vi "五层电梯.vi"() -> ()   [LabVIEW 2011]
panel:
  in  "上/下行显示":string
  in  "楼层显示":string
  out "电梯内厢显示":string
  out "5层显示":string
  out "4层显示":string
  out "3层显示":string
  out "2层显示":string
  out "1层显示":string
  in  "上/下行控制":i32
  out "内外呼叫数组":bool[](array[boolean])
  out "电梯门":bool
  in  "内呼1层":bool caption="1"
  in  "内呼2层":bool caption="2"
  in  "内呼3层":bool caption="3"
  in  "内呼4层":bool caption="4"
  in  "内呼5层":bool caption="5"
  in  "5下":bool caption="下"
  in  "1上":bool caption="上"
  in  "4下":bool caption="下"
  in  "4上":bool caption="上"
  in  "3下":bool caption="下"
  in  "3上":bool caption="上"
  in  "2下":bool caption="下"
  in  "2上":bool caption="上"
  out "五层门":bool caption="Boolean"
  out "四层门":bool caption="Boolean"
  out "三层门":bool caption="Boolean"
  out "二层门":bool caption="Boolean"
  out "一层门":bool caption="Boolean"
  out "电梯":bool
  # "五层电梯示意图"
  # "5"
  # "4"
  # "3"
  # "电梯内厢"
  # "2"
  # "1"
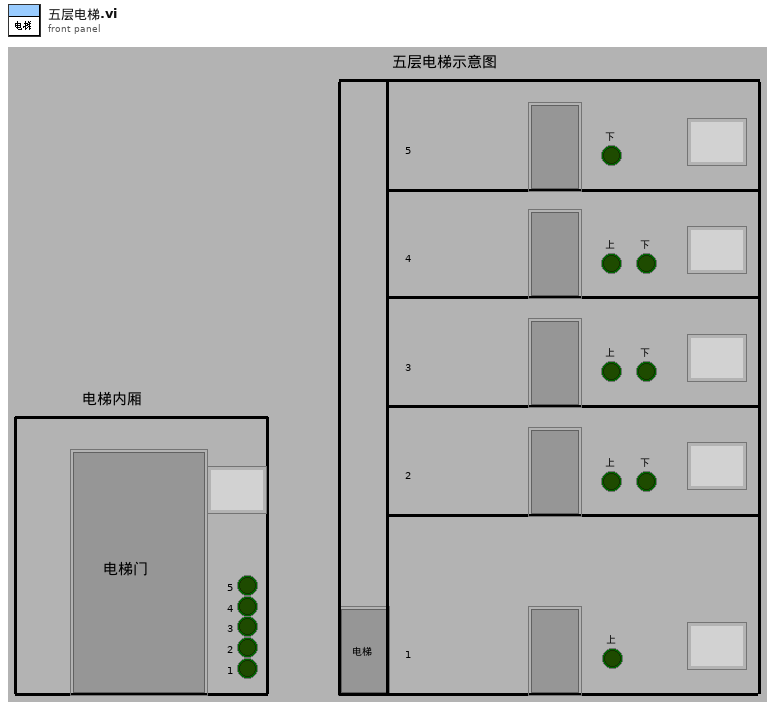
[diagram p1: front panel]
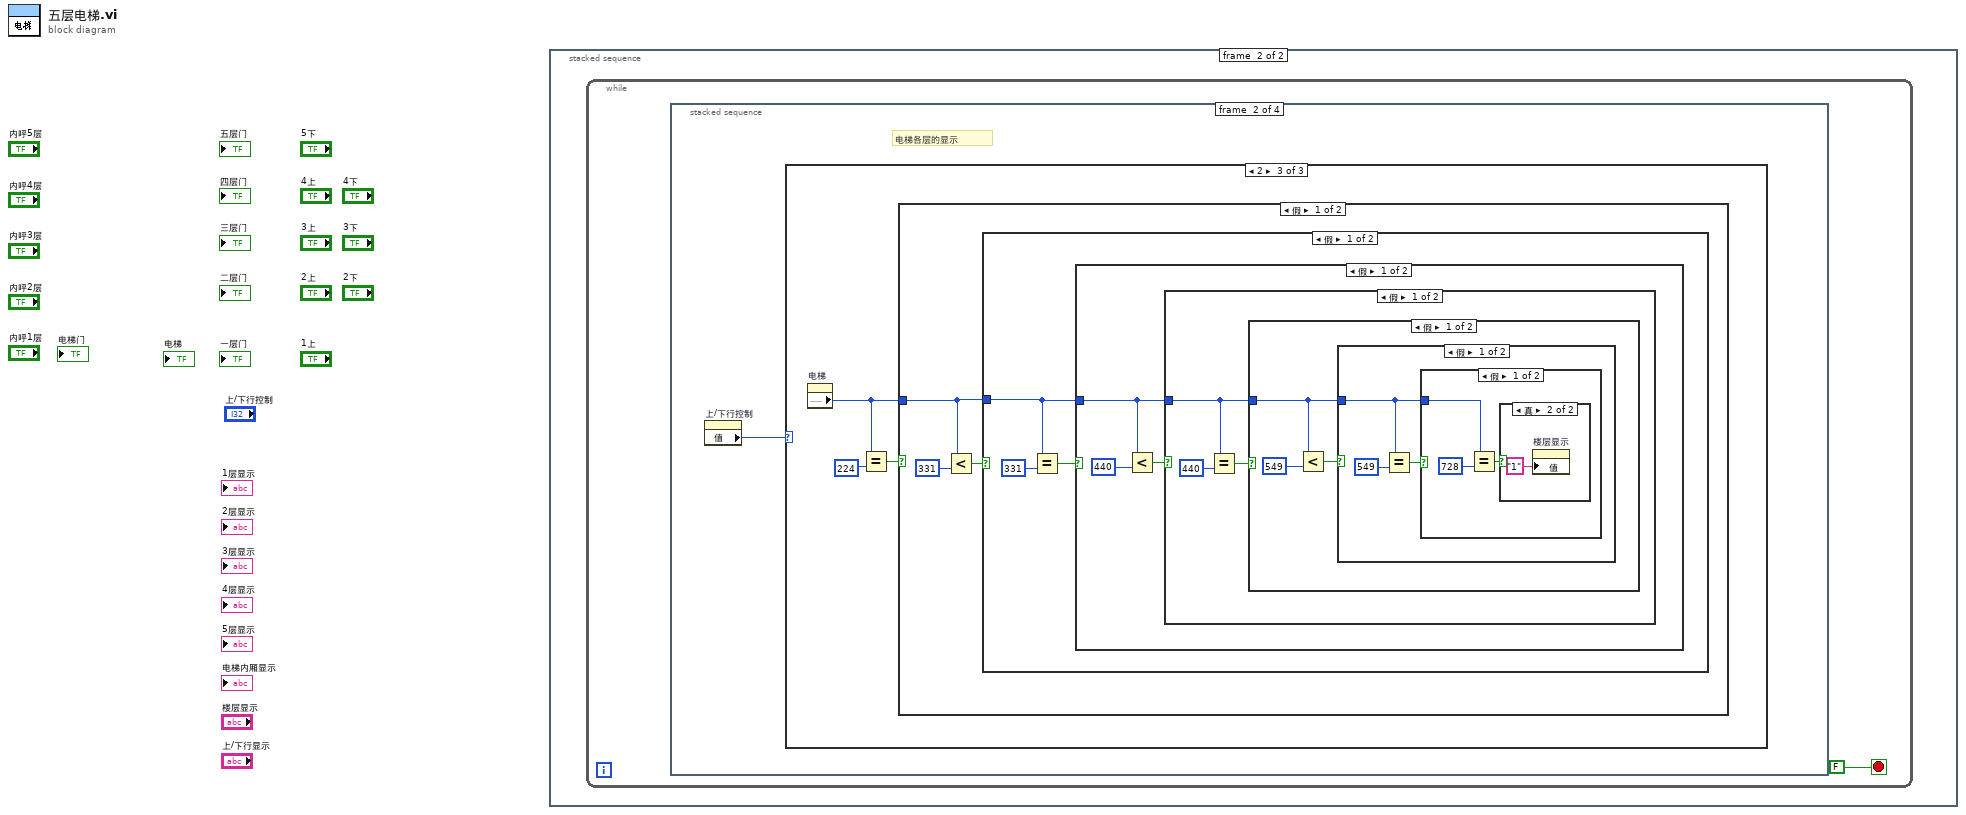
[diagram p0: block diagram]
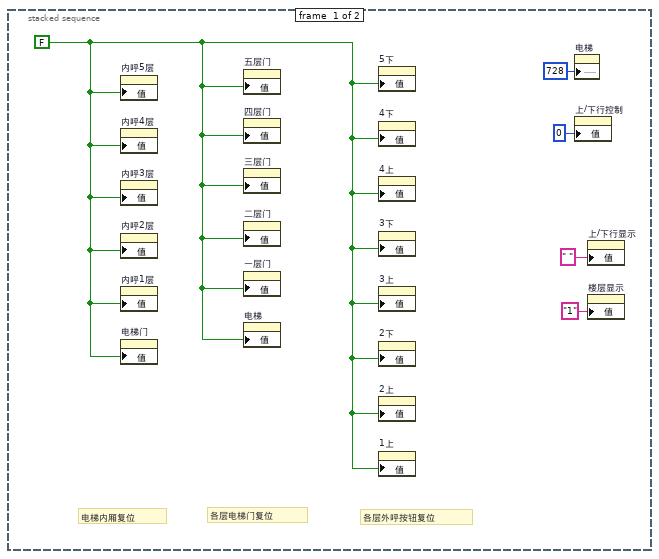
[diagram p2: hidden frame]
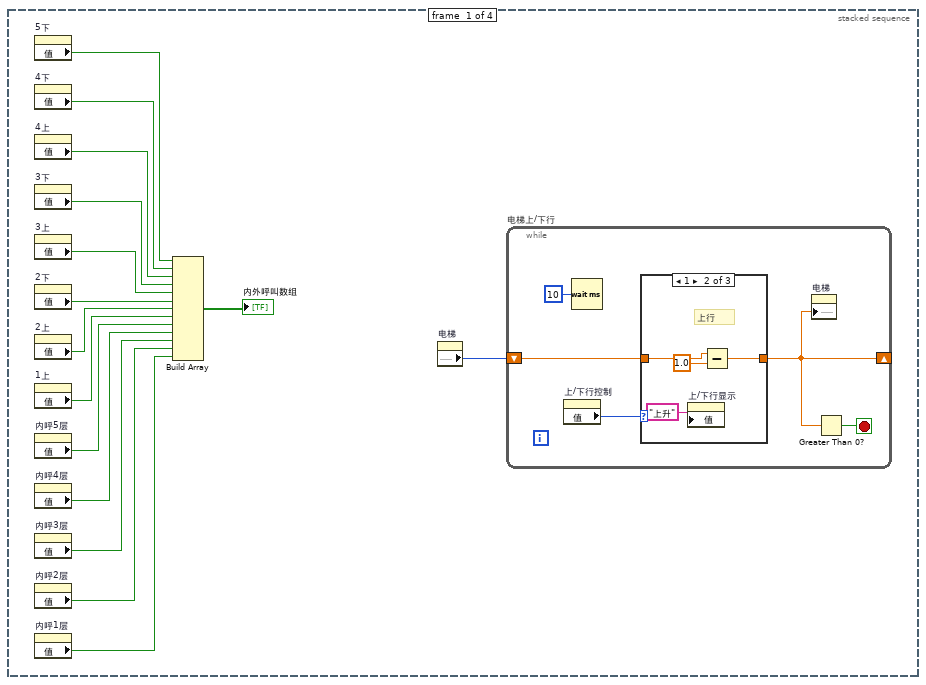
[diagram p3: hidden frame]
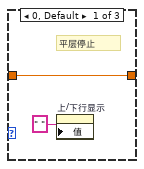
[diagram p4: hidden frame]
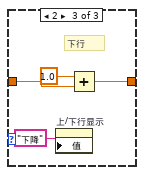
[diagram p5: hidden frame]
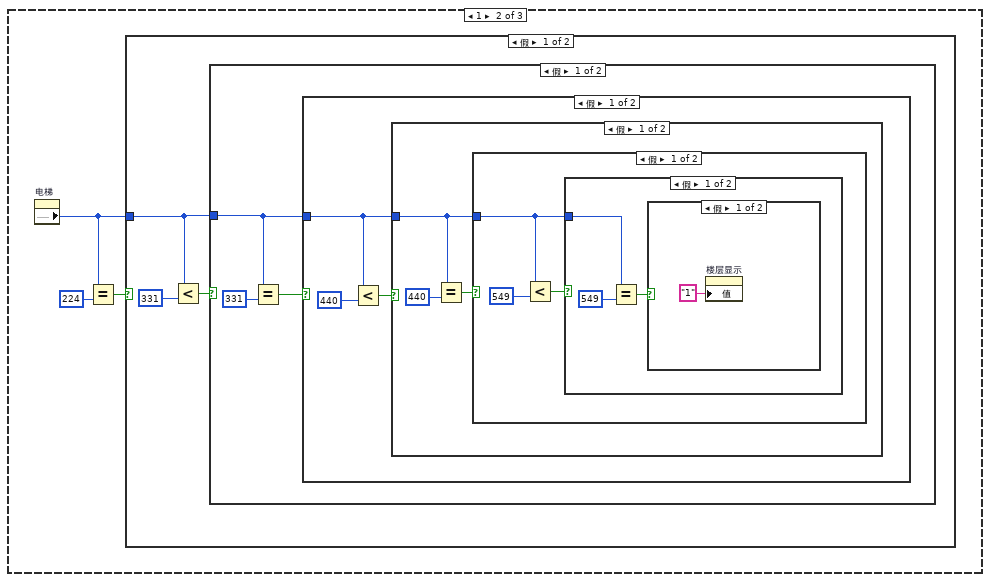
[diagram p7: hidden frame]
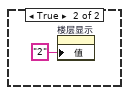
[diagram p8: hidden frame]
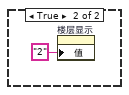
[diagram p9: hidden frame]
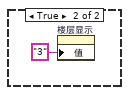
[diagram p10: hidden frame]
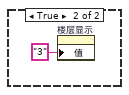
[diagram p11: hidden frame]
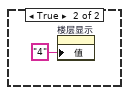
[diagram p12: hidden frame]
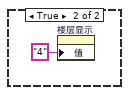
[diagram p13: hidden frame]
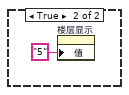
[diagram p14: hidden frame]
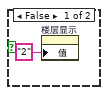
[diagram p15: hidden frame]
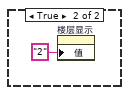
[diagram p16: hidden frame]
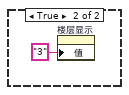
[diagram p17: hidden frame]
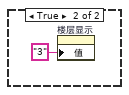
[diagram p18: hidden frame]
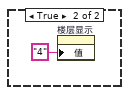
[diagram p19: hidden frame]
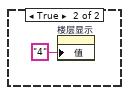
[diagram p20: hidden frame]
diagram:
  n1 = stacked-sequence {
    frame #0 {
      w3 = FALSE ("开门")
      # "各层外呼按钮复位"
      # "各层电梯门复位"
      # "电梯内厢复位"
      n2 = property on="内呼5层" class="Bool (严格)"("值"=w3) -> ()  [unwired: 2 in, 2 out]
      n3 = property on="内呼4层" class="Bool (严格)"("值"=w3) -> ()  [unwired: 2 in, 2 out]
      n4 = property on="内呼3层" class="Bool (严格)"("值"=w3) -> ()  [unwired: 2 in, 2 out]
      n5 = property on="内呼2层" class="Bool (严格)"("值"=w3) -> ()  [unwired: 2 in, 2 out]
      n6 = property on="内呼1层" class="Bool (严格)"("值"=w3) -> ()  [unwired: 2 in, 2 out]
      n7 = property on="电梯门" class="Bool (严格)"("值"=w3) -> ()  [unwired: 2 in, 2 out]
      n8 = property on="五层门" class="Bool (严格)"("值"=w3) -> ()  [unwired: 2 in, 2 out]
      n9 = property on="四层门" class="Bool (严格)"("值"=w3) -> ()  [unwired: 2 in, 2 out]
      n10 = property on="三层门" class="Bool (严格)"("值"=w3) -> ()  [unwired: 2 in, 2 out]
      n11 = property on="二层门" class="Bool (严格)"("值"=w3) -> ()  [unwired: 2 in, 2 out]
      n12 = property on="一层门" class="Bool (严格)"("值"=w3) -> ()  [unwired: 2 in, 2 out]
      n13 = property on="电梯" class="Bool (严格)"("值"=w3) -> ()  [unwired: 2 in, 2 out]
      n14 = property on="5下" class="Bool (严格)"("值"=w3) -> ()  [unwired: 2 in, 2 out]
      n15 = property on="4下" class="Bool (严格)"("值"=w3) -> ()  [unwired: 2 in, 2 out]
      n16 = property on="4上" class="Bool (严格)"("值"=w3) -> ()  [unwired: 2 in, 2 out]
      n17 = property on="3下" class="Bool (严格)"("值"=w3) -> ()  [unwired: 2 in, 2 out]
      n18 = property on="3上" class="Bool (严格)"("值"=w3) -> ()  [unwired: 2 in, 2 out]
      n19 = property on="2下" class="Bool (严格)"("值"=w3) -> ()  [unwired: 2 in, 2 out]
      n20 = property on="2上" class="Bool (严格)"("值"=w3) -> ()  [unwired: 2 in, 2 out]
      n21 = property on="1上" class="Bool (严格)"("值"=w3) -> ()  [unwired: 2 in, 2 out]
      n22 = property on="电梯" class="Bool (严格)"("位置:置顶"=728 ("Position:Top")) -> ()  [unwired: 2 in, 2 out]
      n23 = property on="上/下行控制" class="DigNum (严格)"("值"=0 ("上/下行控制")) -> ()  [unwired: 2 in, 2 out]
      n24 = property on="上/下行显示" class="Str"("值"=" " ("上/下行显示")) -> ()  [unwired: 2 in, 2 out]
      n25 = property on="楼层显示" class="Str"("值"="1" ("楼层显示")) -> ()  [unwired: 2 in, 2 out]
    }
    frame #1 {
      n26 = while {
        stop <- FALSE stop-if-true
        n27 = stacked-sequence {
          frame #0 {
            n28 = property on="5下" class="Bool (严格)"() -> ("值"=w20:bool)  [unwired: 2 in, 2 out]
            n29 = property on="4下" class="Bool (严格)"() -> ("值"=w19:bool)  [unwired: 2 in, 2 out]
            n30 = property on="4上" class="Bool (严格)"() -> ("值"=w18:bool)  [unwired: 2 in, 2 out]
            n31 = property on="3下" class="Bool (严格)"() -> ("值"=w17:bool)  [unwired: 2 in, 2 out]
            n32 = property on="3上" class="Bool (严格)"() -> ("值"=w16:bool)  [unwired: 2 in, 2 out]
            n33 = property on="2下" class="Bool (严格)"() -> ("值"=w15:bool)  [unwired: 2 in, 2 out]
            n34 = property on="2上" class="Bool (严格)"() -> ("值"=w14:bool)  [unwired: 2 in, 2 out]
            n35 = property on="1上" class="Bool (严格)"() -> ("值"=w13:bool)  [unwired: 2 in, 2 out]
            n36 = property on="内呼5层" class="Bool (严格)"() -> ("值"=w12:bool)  [unwired: 2 in, 2 out]
            n37 = property on="内呼4层" class="Bool (严格)"() -> ("值"=w11:bool)  [unwired: 2 in, 2 out]
            n38 = property on="内呼3层" class="Bool (严格)"() -> ("值"=w10:bool)  [unwired: 2 in, 2 out]
            n39 = property on="内呼2层" class="Bool (严格)"() -> ("值"=w9:bool)  [unwired: 2 in, 2 out]
            n40 = property on="内呼1层" class="Bool (严格)"() -> ("值"=w8:bool)  [unwired: 2 in, 2 out]
            n41 = Build Array(w20, w19, w18, w17, w16, w15, w14, w13, w12, w11, w10, w9, w8) -> (→"内外呼叫数组":bool[])
            n42 = property on="电梯" class="Bool (严格)"() -> ("位置:置顶"=w21:i32)  [unwired: 2 in, 2 out]
            n43 = while "电梯上/下行" {
              shift-right: [w23] -> _
              shift-left: w21 -> [w24]
              stop <- w22 stop-if-true
              n44 = property on="上/下行控制" class="DigNum (严格)"() -> ("值"=w25:i32)  [unwired: 2 in, 2 out]
              n45 = Wait (ms)(milliseconds to wait=u32 10) -> ()  [unwired: 1 out]
              n46 = case shown="1" w25 {
                tunnel: w24 -> [w28 w31 w36]
                tunnel: [w28 w32 w35] -> w23
                frame 0, Default {
                  # "平层停止"
                  n47 = property on="上/下行显示" class="Str"("值"=" " ("上/下行显示")) -> ()  [unwired: 2 in, 2 out]
                }
                frame 1 {
                  # "上行"
                  n48 = property on="上/下行显示" class="Str"("值"="上升" ("上/下行显示")) -> ()  [unwired: 2 in, 2 out]
                  n49 = Subtract(x=w31, y=1.0) -> (x-y=w32:dbl)
                }
                frame 2 {
                  # "下行"
                  n50 = property on="上/下行显示" class="Str"("值"="下降" ("上/下行显示")) -> ()  [unwired: 2 in, 2 out]
                  n51 = Add(x=1.0, y=w36) -> (x+y=w35:dbl)
                }
              }
              n52 = property on="电梯" class="Bool (严格)"("位置:置顶"=w23) -> ()  [unwired: 2 in, 2 out]
              n53 = Greater Than 0?(x=w23) -> (x > 0?=w22:bool)
            }
          }
          frame #1 {
            # "电梯各层的显示"
            n54 = property on="上/下行控制" class="DigNum (严格)"() -> ("值"=w37:i32)  [unwired: 2 in, 2 out]
            n55 = case shown="2" w37 {
              frame 0, Default {
              }
              frame 1 {
                n56 = property on="电梯" class="Bool (严格)"() -> ("位置:置顶"=w38:i32)  [unwired: 2 in, 2 out]
                n57 = Equal?(x=w38, y=224) -> (x = y?=w39:bool)
                n58 = case shown="假" w39 {
                  tunnel: w38 -> [w41 _]
                  frame False {
                    n59 = Less?(x=w41, y=331) -> (x < y?=w42:bool)
                    n60 = case shown="假" w42 {
                      tunnel: w41 -> [w44 _]
                      frame False {
                        n61 = Equal?(x=w44, y=331) -> (x = y?=w45:bool)
                        n62 = case shown="假" w45 {
                          tunnel: w44 -> [w47 _]
                          frame False {
                            n63 = Less?(x=w47, y=440) -> (x < y?=w48:bool)
                            n64 = case shown="假" w48 {
                              tunnel: w47 -> [w50 _]
                              frame False {
                                n65 = Equal?(x=w50, y=440) -> (x = y?=w51:bool)
                                n66 = case shown="假" w51 {
                                tunnel: w50 -> [w53 _]
                                frame False {
                                n67 = Less?(x=w53, y=549) -> (x < y?=w54:bool)
                                n68 = case shown="假" w54 {
                                tunnel: w53 -> [w57 _]
                                frame False {
                                n69 = Equal?(x=w57, y=549) -> (x = y?=w56:bool)
                                n70 = case shown="假" w56 {
                                frame False {
                                n71 = property on="楼层显示" class="Str"("值"="1" ("楼层显示")) -> ()  [unwired: 2 in, 2 out]
                                }
                                frame True {
                                n72 = property on="楼层显示" class="Str"("值"="2" ("楼层显示")) -> ()  [unwired: 2 in, 2 out]
                                }
                                }
                                }
                                frame True {
                                n73 = property on="楼层显示" class="Str"("值"="2" ("楼层显示")) -> ()  [unwired: 2 in, 2 out]
                                }
                                }
                                }
                                frame True {
                                n74 = property on="楼层显示" class="Str"("值"="3" ("楼层显示")) -> ()  [unwired: 2 in, 2 out]
                                }
                                }
                              }
                              frame True {
                                n75 = property on="楼层显示" class="Str"("值"="3" ("楼层显示")) -> ()  [unwired: 2 in, 2 out]
                              }
                            }
                          }
                          frame True {
                            n76 = property on="楼层显示" class="Str"("值"="4" ("楼层显示")) -> ()  [unwired: 2 in, 2 out]
                          }
                        }
                      }
                      frame True {
                        n77 = property on="楼层显示" class="Str"("值"="4" ("楼层显示")) -> ()  [unwired: 2 in, 2 out]
                      }
                    }
                  }
                  frame True {
                    n78 = property on="楼层显示" class="Str"("值"="5" ("楼层显示")) -> ()  [unwired: 2 in, 2 out]
                  }
                }
              }
              frame 2 {
                n79 = property on="电梯" class="Bool (严格)"() -> ("位置:置顶"=w67:i32)  [unwired: 2 in, 2 out]
                n80 = Equal?(x=w67, y=224) -> (x = y?=w68:bool)
                n81 = case shown="假" w68 {
                  tunnel: w67 -> [w70 _]
                  frame False {
                    n82 = Less?(x=w70, y=331) -> (x < y?=w71:bool)
                    n83 = case shown="假" w71 {
                      tunnel: w70 -> [w73 _]
                      frame False {
                        n84 = Equal?(x=w73, y=331) -> (x = y?=w74:bool)
                        n85 = case shown="假" w74 {
                          tunnel: w73 -> [w76 _]
                          frame False {
                            n86 = Less?(x=w76, y=440) -> (x < y?=w77:bool)
                            n87 = case shown="假" w77 {
                              tunnel: w76 -> [w79 _]
                              frame False {
                                n88 = Equal?(x=w79, y=440) -> (x = y?=w80:bool)
                                n89 = case shown="假" w80 {
                                tunnel: w79 -> [w82 _]
                                frame False {
                                n90 = Less?(x=w82, y=549) -> (x < y?=w83:bool)
                                n91 = case shown="假" w83 {
                                tunnel: w82 -> [w85 _]
                                frame False {
                                n92 = Equal?(x=w85, y=549) -> (x = y?=w86:bool)
                                n93 = case shown="假" w86 {
                                tunnel: w85 -> [w89 _]
                                frame False {
                                n94 = Equal?(x=w89, y=728) -> (x = y?=w88:bool)
                                n95 = case shown="真" w88 {
                                frame False {
                                n96 = property on="楼层显示" class="Str"("值"="2" ("楼层显示")) -> ()  [unwired: 2 in, 2 out]
                                }
                                frame True {
                                n97 = property on="楼层显示" class="Str"("值"="1" ("楼层显示")) -> ()  [unwired: 2 in, 2 out]
                                }
                                }
                                }
                                frame True {
                                n98 = property on="楼层显示" class="Str"("值"="2" ("楼层显示")) -> ()  [unwired: 2 in, 2 out]
                                }
                                }
                                }
                                frame True {
                                n99 = property on="楼层显示" class="Str"("值"="3" ("楼层显示")) -> ()  [unwired: 2 in, 2 out]
                                }
                                }
                                }
                                frame True {
                                n100 = property on="楼层显示" class="Str"("值"="3" ("楼层显示")) -> ()  [unwired: 2 in, 2 out]
                                }
                                }
                              }
                              frame True {
                                n101 = property on="楼层显示" class="Str"("值"="4" ("楼层显示")) -> ()  [unwired: 2 in, 2 out]
                              }
                            }
                          }
                          frame True {
                            n102 = property on="楼层显示" class="Str"("值"="4" ("楼层显示")) -> ()  [unwired: 2 in, 2 out]
                          }
                        }
                      }
                      frame True {
                        n103 = property on="楼层显示" class="Str"("值"="5" ("楼层显示")) -> ()  [unwired: 2 in, 2 out]
                      }
                    }
                  }
                  frame True {
                    n104 = property on="楼层显示" class="Str"("值"="5" ("楼层显示")) -> ()  [unwired: 2 in, 2 out]
                  }
                }
              }
            }
          }
          frame #2 {
            n105 = property on="上/下行显示" class="Str"() -> ("值"=w101:string)  [unwired: 2 in, 2 out]
            n106 = property on="楼层显示" class="Str"() -> ("值"=w103:string)  [unwired: 2 in, 2 out]
            n107 = Concatenate Strings(w101, "\r", w103) -> (w100:string)
            n108 = property on="1层显示" class="Str"("值"=w100) -> ()  [unwired: 2 in, 2 out]
            n109 = property on="2层显示" class="Str"("值"=w100) -> ()  [unwired: 2 in, 2 out]
            n110 = property on="3层显示" class="Str"("值"=w100) -> ()  [unwired: 2 in, 2 out]
            n111 = property on="4层显示" class="Str"("值"=w100) -> ()  [unwired: 2 in, 2 out]
            n112 = property on="5层显示" class="Str"("值"=w100) -> ()  [unwired: 2 in, 2 out]
            n113 = property on="电梯内厢显示" class="Str"("值"=w100) -> ()  [unwired: 2 in, 2 out]
          }
          frame #3 {
            n114 = property on="电梯" class="Bool (严格)"() -> ("位置:置顶"=w104:i32)  [unwired: 2 in, 2 out]
            n115 = case shown="440" w104 {
              frame 0, Default {
              }
              frame 728 {
                # "一层动作"
                n116 = stacked-sequence {
                  frame #0 {
                    n117 = property on="内呼1层" class="Bool (严格)"() -> ("值"=w107:bool)  [unwired: 2 in, 2 out]
                    n118 = property on="1上" class="Bool (严格)"() -> ("值"=w106:bool)  [unwired: 2 in, 2 out]
                    n119 = Or(x=w107, y=w106) -> (x .or. y?=w105:bool)
                    n120 = case shown="假" w105 {
                      frame False {
                      }
                      frame True {
                        n121 = stacked-sequence {
                          frame #0 {
                            w108 = TRUE ("一层门")
                            # "开门"
                            n122 = property on="一层门" class="Bool (严格)"("值"=w108) -> ()  [unwired: 2 in, 2 out]
                            n123 = property on="电梯门" class="Bool (严格)"("值"=w108) -> ()  [unwired: 2 in, 2 out]
                          }
                          frame #1 {
                            # "进出电梯延时"
                            n124 = Wait (ms)(milliseconds to wait=u32 3000) -> ()  [unwired: 1 out]
                          }
                          frame #2 {
                            w110 = FALSE ("一层门")
                            # "关门"
                            n125 = property on="内呼1层" class="Bool (严格)"("值"=w110) -> ()  [unwired: 2 in, 2 out]
                            n126 = property on="1上" class="Bool (严格)"("值"=w110) -> ()  [unwired: 2 in, 2 out]
                            n127 = property on="一层门" class="Bool (严格)"("值"=w110) -> ()  [unwired: 2 in, 2 out]
                            n128 = property on="电梯门" class="Bool (严格)"("值"=w110) -> ()  [unwired: 2 in, 2 out]
                          }
                        }
                      }
                    }
                  }
                  frame #1 {
                    n129 = property on="内外呼叫数组" class="Arr (严格)"() -> ("值"=w125:bool[])  [unwired: 2 in, 2 out]
                    n130 = Index Array(array=w125, index #1=0 ("index"), index #8=8 ("index")) -> (element #1=w122:bool, element #2=w121:bool, element #3=w120:bool, element #4=w119:bool, element #5=w118:bool, element #6=w117:bool, element #7=w116:bool, element #8=w115:bool, element #9=w114:bool, element #10=w113:bool, element #11=w112:bool)  [unwired: 9 in]
                    n131 = Build Array(w122, w121, w120, w119, w118, w117, w116, w115, w114, w113, w112) -> (w111:bool[])
                    n132 = Or Array Elements(Boolean array=w111) -> (logical OR=w126:bool)
                    n133 = case shown="真" w126 {
                      frame False {
                        n134 = property on="上/下行控制" class="DigNum (严格)"("值"=0 ("上/下行控制")) -> ()  [unwired: 2 in, 2 out]
                      }
                      frame True {
                        n135 = property on="上/下行控制" class="DigNum (严格)"("值"=1 ("上/下行控制")) -> ()  [unwired: 2 in, 2 out]
                      }
                    }
                  }
                }
              }
              frame 549 {
                # "二层动作"
                n136 = property on="上/下行控制" class="DigNum (严格)"() -> ("值"=w129:i32)  [unwired: 2 in, 2 out]
                n137 = case shown="1" w129 {
                  frame 0, Default {
                    # "从静止到上行，下行，同时响应时采取就近原则"
                    n138 = stacked-sequence {
                      frame #0 {
                        # "二层开关门动作"
                        n139 = property on="内外呼叫数组" class="Arr (严格)"() -> ("值"=w132:bool[])  [unwired: 2 in, 2 out]
                        n140 = Index Array(array=w132, index #1=5 ("index"), index #3=11 ("index")) -> (element #1=w134:bool, element #2=w135:bool, element #3=w136:bool)  [unwired: 1 in]
                        n141 = Build Array(w134, w135, w136) -> (w137:bool[])
                        n142 = Or Array Elements(Boolean array=w137) -> (logical OR=w130:bool)
                        n143 = case shown="真" w130 {
                          frame False {
                          }
                          frame True {
                            n144 = stacked-sequence {
                              frame #0 {
                                w138 = TRUE ("二层门")
                                # "开门"
                                n145 = property on="二层门" class="Bool (严格)"("值"=w138) -> ()  [unwired: 2 in, 2 out]
                                n146 = property on="电梯门" class="Bool (严格)"("值"=w138) -> ()  [unwired: 2 in, 2 out]
                              }
                              frame #1 {
                                # "进出电梯延时"
                                n147 = Wait (ms)(milliseconds to wait=u32 3000) -> ()  [unwired: 1 out]
                              }
                              frame #2 {
                                w140 = FALSE ("二层门")
                                # "关门"
                                n148 = property on="2下" class="Bool (严格)"("值"=w140) -> ()  [unwired: 2 in, 2 out]
                                n149 = property on="二层门" class="Bool (严格)"("值"=w140) -> ()  [unwired: 2 in, 2 out]
                                n150 = property on="电梯门" class="Bool (严格)"("值"=w140) -> ()  [unwired: 2 in, 2 out]
                                n151 = property on="2上" class="Bool (严格)"("值"=w140) -> ()  [unwired: 2 in, 2 out]
                                n152 = property on="内呼2层" class="Bool (严格)"("值"=w140) -> ()  [unwired: 2 in, 2 out]
                              }
                            }
                          }
                        }
                      }
                      frame #1 {
                        n153 = property on="内外呼叫数组" class="Arr (严格)"() -> ("值"=w146:bool[])  [unwired: 2 in, 2 out]
                        n154 = Index Array(array=w146, index #1=0 ("index"), index #6=8 ("index")) -> (element #1=w148:bool, element #2=w149:bool, element #3=w150:bool, element #4=w151:bool, element #5=w152:bool, element #6=w143:bool, element #7=w142:bool, element #8=w141:bool)  [unwired: 6 in]
                        n155 = Build Array(w148, w149, w150, w151, w152, w143, w142, w141) -> (w153:bool[])
                        n156 = Or Array Elements(Boolean array=w153) -> (logical OR=w145:bool)
                        n157 = case shown="真" w145 {
                          frame False {
                          }
                          frame True {
                            n158 = property on="上/下行控制" class="DigNum (严格)"("值"=1 ("上/下行控制")) -> ()  [unwired: 2 in, 2 out]
                          }
                        }
                      }
                      frame #2 {
                        n159 = property on="1上" class="Bool (严格)"() -> ("值"=w157:bool)  [unwired: 2 in, 2 out]
                        n160 = property on="内呼1层" class="Bool (严格)"() -> ("值"=w156:bool)  [unwired: 2 in, 2 out]
                        n161 = Or(x=w157, y=w156) -> (x .or. y?=w155:bool)
                        n162 = case shown="真" w155 {
                          frame False {
                          }
                          frame True {
                            n163 = property on="上/下行控制" class="DigNum (严格)"("值"=2 ("上/下行控制")) -> ()  [unwired: 2 in, 2 out]
                          }
                        }
                      }
                    }
                  }
                  frame 1 {
                    n164 = property on="内外呼叫数组" class="Arr (严格)"() -> ("值"=w171:bool[])  [unwired: 2 in, 2 out]
                    n165 = Index Array(array=w171, index #1=0 ("index"), index #6=8 ("index")) -> (element #1=w169:bool, element #2=w168:bool, element #3=w167:bool, element #4=w166:bool, element #5=w165:bool, element #6=w161:bool, element #7=w160:bool, element #8=w159:bool)  [unwired: 6 in]
                    n166 = Build Array(w169, w168, w167, w166, w165, w161, w160, w159) -> (w164:bool[])
                    n167 = Or Array Elements(Boolean array=w164) -> (logical OR=w163:bool)
                    n168 = case shown="真" w163 {
                      frame False {
                        n169 = stacked-sequence {
                          frame #0 {
                            n170 = property on="2下" class="Bool (严格)"() -> ("值"=w172:bool)  [unwired: 2 in, 2 out]
                            n171 = case shown="真" w172 {
                              frame False {
                              }
                              frame True {
                                n172 = stacked-sequence {
                                frame #0 {
                                w173 = TRUE ("二层门")
                                # "开门"
                                n173 = property on="二层门" class="Bool (严格)"("值"=w173) -> ()  [unwired: 2 in, 2 out]
                                n174 = property on="电梯门" class="Bool (严格)"("值"=w173) -> ()  [unwired: 2 in, 2 out]
                                }
                                frame #1 {
                                # "进出电梯延时"
                                n175 = Wait (ms)(milliseconds to wait=u32 3000) -> ()  [unwired: 1 out]
                                }
                                frame #2 {
                                w175 = FALSE ("二层门")
                                # "关门"
                                n176 = property on="二层门" class="Bool (严格)"("值"=w175) -> ()  [unwired: 2 in, 2 out]
                                n177 = property on="电梯门" class="Bool (严格)"("值"=w175) -> ()  [unwired: 2 in, 2 out]
                                n178 = property on="2下" class="Bool (严格)"("值"=w175) -> ()  [unwired: 2 in, 2 out]
                                }
                                }
                              }
                            }
                          }
                          frame #1 {
                            n179 = property on="上/下行控制" class="DigNum (严格)"("值"=0 ("上/下行控制")) -> ()  [unwired: 2 in, 2 out]
                          }
                        }
                      }
                      frame True {
                        n180 = property on="2上" class="Bool (严格)"() -> ("值"=w179:bool)  [unwired: 2 in, 2 out]
                        n181 = property on="内呼2层" class="Bool (严格)"() -> ("值"=w178:bool)  [unwired: 2 in, 2 out]
                        n182 = Or(x=w179, y=w178) -> (x .or. y?=w177:bool)
                        n183 = case shown="假" w177 {
                          frame False {
                            n184 = property on="上/下行控制" class="DigNum (严格)"("值"=1 ("上/下行控制")) -> ()  [unwired: 2 in, 2 out]
                          }
                          frame True {
                            n185 = stacked-sequence {
                              frame #0 {
                                w181 = TRUE ("二层门")
                                # "开门"
                                n186 = property on="二层门" class="Bool (严格)"("值"=w181) -> ()  [unwired: 2 in, 2 out]
                                n187 = property on="电梯门" class="Bool (严格)"("值"=w181) -> ()  [unwired: 2 in, 2 out]
                              }
                              frame #1 {
                                # "进出电梯延时"
                                n188 = Wait (ms)(milliseconds to wait=u32 3000) -> ()  [unwired: 1 out]
                              }
                              frame #2 {
                                w183 = FALSE ("二层门")
                                # "关门"
                                n189 = property on="二层门" class="Bool (严格)"("值"=w183) -> ()  [unwired: 2 in, 2 out]
                                n190 = property on="电梯门" class="Bool (严格)"("值"=w183) -> ()  [unwired: 2 in, 2 out]
                                n191 = property on="2上" class="Bool (严格)"("值"=w183) -> ()  [unwired: 2 in, 2 out]
                                n192 = property on="内呼2层" class="Bool (严格)"("值"=w183) -> ()  [unwired: 2 in, 2 out]
                              }
                              frame #3 {
                                n193 = property on="上/下行控制" class="DigNum (严格)"("值"=1 ("上/下行控制")) -> ()  [unwired: 2 in, 2 out]
                              }
                            }
                          }
                        }
                      }
                    }
                  }
                  frame 2 {
                    n194 = property on="1上" class="Bool (严格)"() -> ("值"=w187:bool)  [unwired: 2 in, 2 out]
                    n195 = property on="内呼1层" class="Bool (严格)"() -> ("值"=w186:bool)  [unwired: 2 in, 2 out]
                    n196 = Or(x=w187, y=w186) -> (x .or. y?=w185:bool)
                    n197 = case shown="真" w185 {
                      frame False {
                        n198 = property on="上/下行控制" class="DigNum (严格)"("值"=0 ("上/下行控制")) -> ()  [unwired: 2 in, 2 out]
                      }
                      frame True {
                        n199 = property on="2下" class="Bool (严格)"() -> ("值"=w189:bool)  [unwired: 2 in, 2 out]
                        n200 = property on="内呼2层" class="Bool (严格)"() -> ("值"=w191:bool)  [unwired: 2 in, 2 out]
                        n201 = Or(x=w189, y=w191) -> (x .or. y?=w190:bool)
                        n202 = case shown="真" w190 {
                          frame False {
                            n203 = property on="上/下行控制" class="DigNum (严格)"("值"=2 ("上/下行控制")) -> ()  [unwired: 2 in, 2 out]
                          }
                          frame True {
                            n204 = stacked-sequence {
                              frame #0 {
                                w193 = TRUE ("二层门")
                                # "开门"
                                n205 = property on="二层门" class="Bool (严格)"("值"=w193) -> ()  [unwired: 2 in, 2 out]
                                n206 = property on="电梯门" class="Bool (严格)"("值"=w193) -> ()  [unwired: 2 in, 2 out]
                              }
                              frame #1 {
                                # "进出电梯延时"
                                n207 = Wait (ms)(milliseconds to wait=u32 3000) -> ()  [unwired: 1 out]
                              }
                              frame #2 {
                                w195 = FALSE ("二层门")
                                # "关门"
                                n208 = property on="二层门" class="Bool (严格)"("值"=w195) -> ()  [unwired: 2 in, 2 out]
                                n209 = property on="电梯门" class="Bool (严格)"("值"=w195) -> ()  [unwired: 2 in, 2 out]
                                n210 = property on="2下" class="Bool (严格)"("值"=w195) -> ()  [unwired: 2 in, 2 out]
                                n211 = property on="内呼2层" class="Bool (严格)"("值"=w195) -> ()  [unwired: 2 in, 2 out]
                              }
                              frame #3 {
                                n212 = property on="上/下行控制" class="DigNum (严格)"("值"=2 ("上/下行控制")) -> ()  [unwired: 2 in, 2 out]
                              }
                            }
                          }
                        }
                      }
                    }
                  }
                }
              }
              frame 440 {
                # "三层动作"
                n213 = property on="上/下行控制" class="DigNum (严格)"() -> ("值"=w197:i32)  [unwired: 2 in, 2 out]
                n214 = case shown="0, 默认" w197 {
                  frame 0, Default {
                    # "从静止到上行，下行，同时响应时采取就近原则"
                    n215 = stacked-sequence {
                      frame #0 {
                        # "三层开关门动作"
                        n216 = property on="内外呼叫数组" class="Arr (严格)"() -> ("值"=w200:bool[])  [unwired: 2 in, 2 out]
                        n217 = Index Array(array=w200, index #1=3 ("index"), index #3=10 ("index")) -> (element #1=w202:bool, element #2=w203:bool, element #3=w204:bool)  [unwired: 1 in]
                        n218 = Build Array(w202, w203, w204) -> (w205:bool[])
                        n219 = Or Array Elements(Boolean array=w205) -> (logical OR=w198:bool)
                        n220 = case shown="真" w198 {
                          frame False {
                          }
                          frame True {
                            n221 = stacked-sequence {
                              frame #0 {
                                w206 = TRUE ("二层门")
                                # "开门"
                                n222 = property on="三层门" class="Bool (严格)"("值"=w206) -> ()  [unwired: 2 in, 2 out]
                                n223 = property on="电梯门" class="Bool (严格)"("值"=w206) -> ()  [unwired: 2 in, 2 out]
                              }
                              frame #1 {
                                # "进出电梯延时"
                                n224 = Wait (ms)(milliseconds to wait=u32 3000) -> ()  [unwired: 1 out]
                              }
                              frame #2 {
                                w208 = FALSE ("二层门")
                                # "关门"
                                n225 = property on="内呼3层" class="Bool (严格)"("值"=w208) -> ()  [unwired: 2 in, 2 out]
                                n226 = property on="三层门" class="Bool (严格)"("值"=w208) -> ()  [unwired: 2 in, 2 out]
                                n227 = property on="电梯门" class="Bool (严格)"("值"=w208) -> ()  [unwired: 2 in, 2 out]
                                n228 = property on="3上" class="Bool (严格)"("值"=w208) -> ()  [unwired: 2 in, 2 out]
                                n229 = property on="3下" class="Bool (严格)"("值"=w208) -> ()  [unwired: 2 in, 2 out]
                              }
                            }
                          }
                        }
                      }
                      frame #1 {
                        n230 = property on="内外呼叫数组" class="Arr (严格)"() -> ("值"=w211:bool[])  [unwired: 2 in, 2 out]
                        n231 = Index Array(array=w211, index #1=0 ("index"), index #4=8 ("index")) -> (element #1=w213:bool, element #2=w214:bool, element #3=w215:bool, element #4=w216:bool, element #5=w217:bool)  [unwired: 3 in]
                        n232 = Build Array(w213, w214, w215, w216, w217) -> (w218:bool[])
                        n233 = Or Array Elements(Boolean array=w218) -> (logical OR=w210:bool)
                        n234 = case shown="真" w210 {
                          frame False {
                          }
                          frame True {
                            n235 = property on="上/下行控制" class="DigNum (严格)"("值"=1 ("上/下行控制")) -> ()  [unwired: 2 in, 2 out]
                          }
                        }
                      }
                      frame #2 {
                        # "三层时，先响应下行"
                        n236 = property on="内外呼叫数组" class="Arr (严格)"() -> ("值"=w222:bool[])  [unwired: 2 in, 2 out]
                        n237 = Index Array(array=w222, index #1=5 ("index"), index #4=11 ("index")) -> (element #1=w224:bool, element #2=w225:bool, element #3=w226:bool, element #4=w227:bool, element #5=w228:bool)  [unwired: 3 in]
                        n238 = Build Array(w224, w225, w226, w227, w228) -> (w229:bool[])
                        n239 = Or Array Elements(Boolean array=w229) -> (logical OR=w220:bool)
                        n240 = case shown="真" w220 {
                          frame False {
                          }
                          frame True {
                            n241 = property on="上/下行控制" class="DigNum (严格)"("值"=2 ("上/下行控制")) -> ()  [unwired: 2 in, 2 out]
                          }
                        }
                      }
                    }
                  }
                  frame 1 {
                    n242 = property on="内外呼叫数组" class="Arr (严格)"() -> ("值"=w240:bool[])  [unwired: 2 in, 2 out]
                    n243 = Index Array(array=w240, index #1=0 ("index"), index #4=8 ("index")) -> (element #1=w238:bool, element #2=w237:bool, element #3=w236:bool, element #4=w235:bool, element #5=w234:bool)  [unwired: 3 in]
                    n244 = Build Array(w238, w237, w236, w235, w234) -> (w233:bool[])
                    n245 = Or Array Elements(Boolean array=w233) -> (logical OR=w232:bool)
                    n246 = case shown="真" w232 {
                      frame False {
                        n247 = stacked-sequence {
                          frame #0 {
                            n248 = property on="3下" class="Bool (严格)"() -> ("值"=w241:bool)  [unwired: 2 in, 2 out]
                            n249 = case shown="真" w241 {
                              frame False {
                              }
                              frame True {
                                n250 = stacked-sequence {
                                frame #0 {
                                w242 = TRUE ("二层门")
                                # "开门"
                                n251 = property on="三层门" class="Bool (严格)"("值"=w242) -> ()  [unwired: 2 in, 2 out]
                                n252 = property on="电梯门" class="Bool (严格)"("值"=w242) -> ()  [unwired: 2 in, 2 out]
                                }
                                frame #1 {
                                # "进出电梯延时"
                                n253 = Wait (ms)(milliseconds to wait=u32 3000) -> ()  [unwired: 1 out]
                                }
                                frame #2 {
                                w244 = FALSE ("二层门")
                                # "关门"
                                n254 = property on="三层门" class="Bool (严格)"("值"=w244) -> ()  [unwired: 2 in, 2 out]
                                n255 = property on="电梯门" class="Bool (严格)"("值"=w244) -> ()  [unwired: 2 in, 2 out]
                                n256 = property on="3下" class="Bool (严格)"("值"=w244) -> ()  [unwired: 2 in, 2 out]
                                }
                                }
                              }
                            }
                          }
                          frame #1 {
                            n257 = property on="上/下行控制" class="DigNum (严格)"("值"=0 ("上/下行控制")) -> ()  [unwired: 2 in, 2 out]
                          }
                        }
                      }
                      frame True {
                        n258 = property on="3上" class="Bool (严格)"() -> ("值"=w247:bool)  [unwired: 2 in, 2 out]
                        n259 = property on="内呼3层" class="Bool (严格)"() -> ("值"=w246:bool)  [unwired: 2 in, 2 out]
                        n260 = Or(x=w247, y=w246) -> (x .or. y?=w248:bool)
                        n261 = case shown="真" w248 {
                          frame False {
                            n262 = property on="上/下行控制" class="DigNum (严格)"("值"=1 ("上/下行控制")) -> ()  [unwired: 2 in, 2 out]
                          }
                          frame True {
                            n263 = stacked-sequence {
                              frame #0 {
                                w250 = TRUE ("二层门")
                                # "开门"
                                n264 = property on="三层门" class="Bool (严格)"("值"=w250) -> ()  [unwired: 2 in, 2 out]
                                n265 = property on="电梯门" class="Bool (严格)"("值"=w250) -> ()  [unwired: 2 in, 2 out]
                              }
                              frame #1 {
                                # "进出电梯延时"
                                n266 = Wait (ms)(milliseconds to wait=u32 3000) -> ()  [unwired: 1 out]
                              }
                              frame #2 {
                                w252 = FALSE ("二层门")
                                # "关门"
                                n267 = property on="三层门" class="Bool (严格)"("值"=w252) -> ()  [unwired: 2 in, 2 out]
                                n268 = property on="电梯门" class="Bool (严格)"("值"=w252) -> ()  [unwired: 2 in, 2 out]
                                n269 = property on="3上" class="Bool (严格)"("值"=w252) -> ()  [unwired: 2 in, 2 out]
                                n270 = property on="内呼3层" class="Bool (严格)"("值"=w252) -> ()  [unwired: 2 in, 2 out]
                              }
                              frame #3 {
                                n271 = property on="上/下行控制" class="DigNum (严格)"("值"=1 ("上/下行控制")) -> ()  [unwired: 2 in, 2 out]
                              }
                            }
                          }
                        }
                      }
                    }
                  }
                  frame 2 {
                    n272 = property on="内外呼叫数组" class="Arr (严格)"() -> ("值"=w256:bool[])  [unwired: 2 in, 2 out]
                    n273 = Index Array(array=w256, index #1=5 ("index"), index #4=11 ("index")) -> (element #1=w258:bool, element #2=w259:bool, element #3=w260:bool, element #4=w261:bool, element #5=w262:bool)  [unwired: 3 in]
                    n274 = Build Array(w258, w259, w260, w261, w262) -> (w263:bool[])
                    n275 = Or Array Elements(Boolean array=w263) -> (logical OR=w254:bool)
                    n276 = case shown="真" w254 {
                      frame False {
                        n277 = property on="上/下行控制" class="DigNum (严格)"("值"=0 ("上/下行控制")) -> ()  [unwired: 2 in, 2 out]
                      }
                      frame True {
                        n278 = property on="3下" class="Bool (严格)"() -> ("值"=w265:bool)  [unwired: 2 in, 2 out]
                        n279 = property on="内呼3层" class="Bool (严格)"() -> ("值"=w267:bool)  [unwired: 2 in, 2 out]
                        n280 = Or(x=w265, y=w267) -> (x .or. y?=w266:bool)
                        n281 = case shown="真" w266 {
                          frame False {
                            n282 = property on="上/下行控制" class="DigNum (严格)"("值"=2 ("上/下行控制")) -> ()  [unwired: 2 in, 2 out]
                          }
                          frame True {
                            n283 = stacked-sequence {
                              frame #0 {
                                w269 = TRUE ("二层门")
                                # "开门"
                                n284 = property on="电梯门" class="Bool (严格)"("值"=w269) -> ()  [unwired: 2 in, 2 out]
                                n285 = property on="三层门" class="Bool (严格)"("值"=w269) -> ()  [unwired: 2 in, 2 out]
                              }
                              frame #1 {
                                # "进出电梯延时"
                                n286 = Wait (ms)(milliseconds to wait=u32 3000) -> ()  [unwired: 1 out]
                              }
                              frame #2 {
                                w271 = FALSE ("二层门")
                                # "关门"
                                n287 = property on="3下" class="Bool (严格)"("值"=w271) -> ()  [unwired: 2 in, 2 out]
                                n288 = property on="电梯门" class="Bool (严格)"("值"=w271) -> ()  [unwired: 2 in, 2 out]
                                n289 = property on="三层门" class="Bool (严格)"("值"=w271) -> ()  [unwired: 2 in, 2 out]
                                n290 = property on="内呼3层" class="Bool (严格)"("值"=w271) -> ()  [unwired: 2 in, 2 out]
                              }
                              frame #3 {
                                n291 = property on="上/下行控制" class="DigNum (严格)"("值"=2 ("上/下行控制")) -> ()  [unwired: 2 in, 2 out]
                              }
                            }
                          }
                        }
                      }
                    }
                  }
                }
              }
              frame 331 {
                # "四层动作"
                n292 = property on="上/下行控制" class="DigNum (严格)"() -> ("值"=w273:i32)  [unwired: 2 in, 2 out]
                n293 = case shown="2" w273 {
                  frame 0, Default {
                    # "从静止到上行，下行，同时响应时采取就近原则"
                    n294 = stacked-sequence {
                      frame #0 {
                        # "四层开关门动作"
                        n295 = property on="内外呼叫数组" class="Arr (严格)"() -> ("值"=w276:bool[])  [unwired: 2 in, 2 out]
                        n296 = Index Array(array=w276, index #1=1 ("index"), index #3=9 ("index")) -> (element #1=w278:bool, element #2=w279:bool, element #3=w280:bool)  [unwired: 1 in]
                        n297 = Build Array(w278, w279, w280) -> (w281:bool[])
                        n298 = Or Array Elements(Boolean array=w281) -> (logical OR=w274:bool)
                        n299 = case shown="真" w274 {
                          frame False {
                          }
                          frame True {
                            n300 = stacked-sequence {
                              frame #0 {
                                w282 = TRUE ("二层门")
                                # "开门"
                                n301 = property on="电梯门" class="Bool (严格)"("值"=w282) -> ()  [unwired: 2 in, 2 out]
                                n302 = property on="四层门" class="Bool (严格)"("值"=w282) -> ()  [unwired: 2 in, 2 out]
                              }
                              frame #1 {
                                # "进出电梯延时"
                                n303 = Wait (ms)(milliseconds to wait=u32 3000) -> ()  [unwired: 1 out]
                              }
                              frame #2 {
                                w284 = FALSE ("二层门")
                                # "关门"
                                n304 = property on="内呼4层" class="Bool (严格)"("值"=w284) -> ()  [unwired: 2 in, 2 out]
                                n305 = property on="四层门" class="Bool (严格)"("值"=w284) -> ()  [unwired: 2 in, 2 out]
                                n306 = property on="电梯门" class="Bool (严格)"("值"=w284) -> ()  [unwired: 2 in, 2 out]
                                n307 = property on="4上" class="Bool (严格)"("值"=w284) -> ()  [unwired: 2 in, 2 out]
                                n308 = property on="4下" class="Bool (严格)"("值"=w284) -> ()  [unwired: 2 in, 2 out]
                              }
                            }
                          }
                        }
                      }
                      frame #1 {
                        n309 = property on="内外呼叫数组" class="Arr (严格)"() -> ("值"=w290:bool[])  [unwired: 2 in, 2 out]
                        n310 = Index Array(array=w290, index #1=3 ("index"), index #6=10 ("index")) -> (element #1=w292:bool, element #2=w293:bool, element #3=w294:bool, element #4=w295:bool, element #5=w296:bool, element #6=w287:bool, element #7=w286:bool, element #8=w285:bool)  [unwired: 6 in]
                        n311 = Build Array(w292, w293, w294, w295, w296, w287, w286, w285) -> (w297:bool[])
                        n312 = Or Array Elements(Boolean array=w297) -> (logical OR=w289:bool)
                        n313 = case shown="真" w289 {
                          frame False {
                          }
                          frame True {
                            n314 = property on="上/下行控制" class="DigNum (严格)"("值"=2 ("上/下行控制")) -> ()  [unwired: 2 in, 2 out]
                          }
                        }
                      }
                      frame #2 {
                        n315 = property on="内呼5层" class="Bool (严格)"() -> ("值"=w300:bool)  [unwired: 2 in, 2 out]
                        n316 = property on="5下" class="Bool (严格)"() -> ("值"=w301:bool)  [unwired: 2 in, 2 out]
                        n317 = Or(x=w301, y=w300) -> (x .or. y?=w299:bool)
                        n318 = case shown="真" w299 {
                          frame False {
                          }
                          frame True {
                            n319 = property on="上/下行控制" class="DigNum (严格)"("值"=1 ("上/下行控制")) -> ()  [unwired: 2 in, 2 out]
                          }
                        }
                      }
                    }
                  }
                  frame 1 {
                    n320 = property on="内外呼叫数组" class="Arr (严格)"() -> ("值"=w309:bool[])  [unwired: 2 in, 2 out]
                    n321 = Index Array(array=w309, index #1=0 ("index"), index #2=8 ("index")) -> (element #1=w307:bool, element #2=w306:bool)
                    n322 = Build Array(w307, w306) -> (w305:bool[])
                    n323 = Or Array Elements(Boolean array=w305) -> (logical OR=w304:bool)
                    n324 = case shown="真" w304 {
                      frame False {
                        n325 = stacked-sequence {
                          frame #0 {
                            n326 = property on="4下" class="Bool (严格)"() -> ("值"=w310:bool)  [unwired: 2 in, 2 out]
                            n327 = case shown="真" w310 {
                              frame False {
                              }
                              frame True {
                                n328 = stacked-sequence {
                                frame #0 {
                                w311 = TRUE ("二层门")
                                # "开门"
                                n329 = property on="电梯门" class="Bool (严格)"("值"=w311) -> ()  [unwired: 2 in, 2 out]
                                n330 = property on="四层门" class="Bool (严格)"("值"=w311) -> ()  [unwired: 2 in, 2 out]
                                }
                                frame #1 {
                                # "进出电梯延时"
                                n331 = Wait (ms)(milliseconds to wait=u32 3000) -> ()  [unwired: 1 out]
                                }
                                frame #2 {
                                w313 = FALSE ("二层门")
                                # "关门"
                                n332 = property on="电梯门" class="Bool (严格)"("值"=w313) -> ()  [unwired: 2 in, 2 out]
                                n333 = property on="四层门" class="Bool (严格)"("值"=w313) -> ()  [unwired: 2 in, 2 out]
                                n334 = property on="4下" class="Bool (严格)"("值"=w313) -> ()  [unwired: 2 in, 2 out]
                                }
                                }
                              }
                            }
                          }
                          frame #1 {
                            n335 = property on="上/下行控制" class="DigNum (严格)"("值"=0 ("上/下行控制")) -> ()  [unwired: 2 in, 2 out]
                          }
                        }
                      }
                      frame True {
                        n336 = property on="4上" class="Bool (严格)"() -> ("值"=w316:bool)  [unwired: 2 in, 2 out]
                        n337 = property on="内呼4层" class="Bool (严格)"() -> ("值"=w315:bool)  [unwired: 2 in, 2 out]
                        n338 = Or(x=w316, y=w315) -> (x .or. y?=w317:bool)
                        n339 = case shown="真" w317 {
                          frame False {
                            n340 = property on="上/下行控制" class="DigNum (严格)"("值"=1 ("上/下行控制")) -> ()  [unwired: 2 in, 2 out]
                          }
                          frame True {
                            n341 = stacked-sequence {
                              frame #0 {
                                w319 = TRUE ("二层门")
                                # "开门"
                                n342 = property on="电梯门" class="Bool (严格)"("值"=w319) -> ()  [unwired: 2 in, 2 out]
                                n343 = property on="四层门" class="Bool (严格)"("值"=w319) -> ()  [unwired: 2 in, 2 out]
                              }
                              frame #1 {
                                # "进出电梯延时"
                                n344 = Wait (ms)(milliseconds to wait=u32 3000) -> ()  [unwired: 1 out]
                              }
                              frame #2 {
                                w321 = FALSE ("二层门")
                                # "关门"
                                n345 = property on="电梯门" class="Bool (严格)"("值"=w321) -> ()  [unwired: 2 in, 2 out]
                                n346 = property on="四层门" class="Bool (严格)"("值"=w321) -> ()  [unwired: 2 in, 2 out]
                                n347 = property on="4上" class="Bool (严格)"("值"=w321) -> ()  [unwired: 2 in, 2 out]
                                n348 = property on="内呼4层" class="Bool (严格)"("值"=w321) -> ()  [unwired: 2 in, 2 out]
                              }
                              frame #3 {
                                n349 = property on="上/下行控制" class="DigNum (严格)"("值"=1 ("上/下行控制")) -> ()  [unwired: 2 in, 2 out]
                              }
                            }
                          }
                        }
                      }
                    }
                  }
                  frame 2 {
                    n350 = property on="内外呼叫数组" class="Arr (严格)"() -> ("值"=w328:bool[])  [unwired: 2 in, 2 out]
                    n351 = Index Array(array=w328, index #1=3 ("index"), index #6=10 ("index")) -> (element #1=w330:bool, element #2=w331:bool, element #3=w332:bool, element #4=w333:bool, element #5=w334:bool, element #6=w325:bool, element #7=w324:bool, element #8=w323:bool)  [unwired: 6 in]
                    n352 = Build Array(w330, w331, w332, w333, w334, w325, w324, w323) -> (w335:bool[])
                    n353 = Or Array Elements(Boolean array=w335) -> (logical OR=w327:bool)
                    n354 = case shown="真" w327 {
                      frame False {
                        n355 = property on="上/下行控制" class="DigNum (严格)"("值"=0 ("上/下行控制")) -> ()  [unwired: 2 in, 2 out]
                      }
                      frame True {
                        n356 = property on="4下" class="Bool (严格)"() -> ("值"=w337:bool)  [unwired: 2 in, 2 out]
                        n357 = property on="内呼4层" class="Bool (严格)"() -> ("值"=w338:bool)  [unwired: 2 in, 2 out]
                        n358 = Or(x=w337, y=w338) -> (x .or. y?=w339:bool)
                        n359 = case shown="真" w339 {
                          frame False {
                          }
                          frame True {
                            n360 = stacked-sequence {
                              frame #0 {
                                w340 = TRUE ("二层门")
                                # "开门"
                                n361 = property on="电梯门" class="Bool (严格)"("值"=w340) -> ()  [unwired: 2 in, 2 out]
                                n362 = property on="四层门" class="Bool (严格)"("值"=w340) -> ()  [unwired: 2 in, 2 out]
                              }
                              frame #1 {
                                # "进出电梯延时"
                                n363 = Wait (ms)(milliseconds to wait=u32 3000) -> ()  [unwired: 1 out]
                              }
                              frame #2 {
                                w342 = FALSE ("二层门")
                                # "关门"
                                n364 = property on="电梯门" class="Bool (严格)"("值"=w342) -> ()  [unwired: 2 in, 2 out]
                                n365 = property on="四层门" class="Bool (严格)"("值"=w342) -> ()  [unwired: 2 in, 2 out]
                                n366 = property on="4下" class="Bool (严格)"("值"=w342) -> ()  [unwired: 2 in, 2 out]
                                n367 = property on="内呼4层" class="Bool (严格)"("值"=w342) -> ()  [unwired: 2 in, 2 out]
                              }
                              frame #3 {
                                n368 = property on="上/下行控制" class="DigNum (严格)"("值"=2 ("上/下行控制")) -> ()  [unwired: 2 in, 2 out]
                              }
                            }
                          }
                        }
                      }
                    }
                  }
                }
              }
              frame 224 {
                # "五层动作"
                n369 = stacked-sequence {
                  frame #0 {
                    n370 = property on="5下" class="Bool (严格)"() -> ("值"=w344:bool)  [unwired: 2 in, 2 out]
                    n371 = property on="内呼5层" class="Bool (严格)"() -> ("值"=w345:bool)  [unwired: 2 in, 2 out]
                    n372 = Or(x=w344, y=w345) -> (x .or. y?=w346:bool)
                    n373 = case shown="假" w346 {
                      frame False {
                      }
                      frame True {
                        n374 = stacked-sequence {
                          frame #0 {
                            w347 = TRUE ("一层门")
                            # "开门"
                            n375 = property on="电梯门" class="Bool (严格)"("值"=w347) -> ()  [unwired: 2 in, 2 out]
                            n376 = property on="五层门" class="Bool (严格)"("值"=w347) -> ()  [unwired: 2 in, 2 out]
                          }
                          frame #1 {
                            # "进出电梯延时"
                            n377 = Wait (ms)(milliseconds to wait=u32 3000) -> ()  [unwired: 1 out]
                          }
                          frame #2 {
                            w349 = FALSE ("一层门")
                            # "关门"
                            n378 = property on="五层门" class="Bool (严格)"("值"=w349) -> ()  [unwired: 2 in, 2 out]
                            n379 = property on="5下" class="Bool (严格)"("值"=w349) -> ()  [unwired: 2 in, 2 out]
                            n380 = property on="内呼5层" class="Bool (严格)"("值"=w349) -> ()  [unwired: 2 in, 2 out]
                            n381 = property on="电梯门" class="Bool (严格)"("值"=w349) -> ()  [unwired: 2 in, 2 out]
                          }
                        }
                      }
                    }
                  }
                  frame #1 {
                    n382 = property on="内外呼叫数组" class="Arr (严格)"() -> ("值"=w364:bool[])  [unwired: 2 in, 2 out]
                    n383 = Index Array(array=w364, index #1=1 ("index"), index #8=9 ("index")) -> (element #1=w361:bool, element #2=w360:bool, element #3=w359:bool, element #4=w358:bool, element #5=w357:bool, element #6=w356:bool, element #7=w355:bool, element #8=w354:bool, element #9=w353:bool, element #10=w352:bool, element #11=w351:bool)  [unwired: 9 in]
                    n384 = Build Array(w361, w360, w359, w358, w357, w356, w355, w354, w353, w352, w351) -> (w350:bool[])
                    n385 = Or Array Elements(Boolean array=w350) -> (logical OR=w365:bool)
                    n386 = case shown="真" w365 {
                      frame False {
                        n387 = property on="上/下行控制" class="DigNum (严格)"("值"=0 ("上/下行控制")) -> ()  [unwired: 2 in, 2 out]
                      }
                      frame True {
                        n388 = property on="上/下行控制" class="DigNum (严格)"("值"=2 ("上/下行控制")) -> ()  [unwired: 2 in, 2 out]
                      }
                    }
                  }
                }
              }
            }
          }
        }
      }
    }
  }
